vi "ReadTCPIP.vi"(3 "error in":errorcluster, 4 "TCP Timeout":i32=500, 5 "bytes to read":i32=-1, 6 "connection ID":refnum<k5>) -> (0 "errorout":errorcluster, 1 "String":string, 2 "connection ID Out":refnum<k5>)   [LabVIEW 2016]
doc: "Reads a message in from a server"
panel:
  # "-1 means read until a blank line"
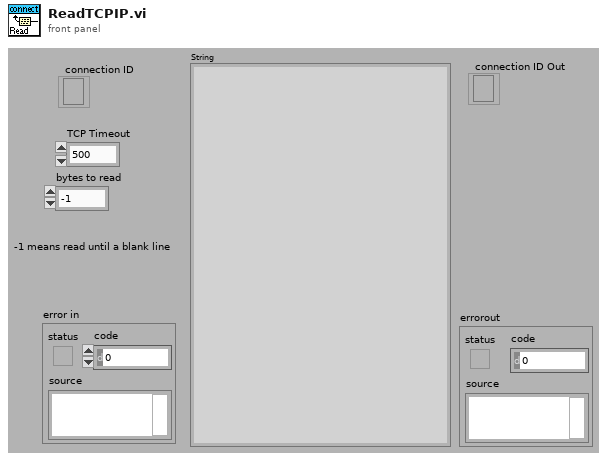
[diagram p1: front panel]
types:
  T1 = enum16{"Standard", "Buffered", "CRLF", "Immediate"}
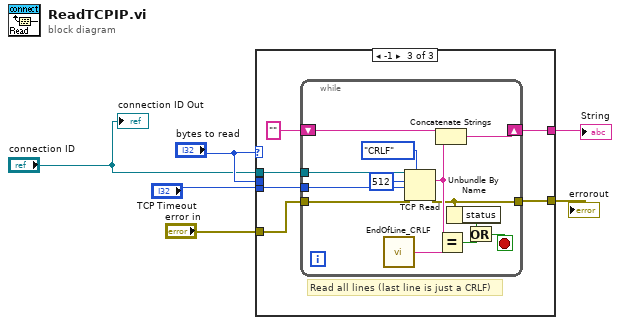
[diagram p0: block diagram]
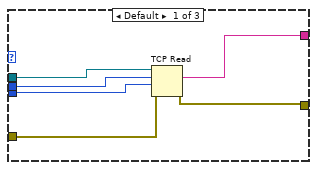
[diagram p2: hidden frame]
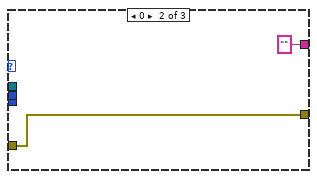
[diagram p3: hidden frame]
diagram:
  n1 = case shown="-1" "bytes to read" {
    tunnel: [w7 "" ("data out") w19] -> w6
    tunnel: [w8 w14 w18] -> w3
    tunnel: "connection ID" -> [w12 _ w17]
    tunnel: "error in" -> [w9 w14 w16]
    tunnel: "TCP Timeout" -> [w10 _ w15]
    tunnel: "bytes to read" -> [w11 _ _]
    frame Default {
      n2 = TCP Read(connection ID=w12, bytes to read=w11, error in (no error)=w9, 9:w10) -> (data out=w7:string, error out=w8:errorcluster)  [unwired: 2 out]
    }
    frame 0 {
    }
    frame -1 {
      # "Read all lines (last line is just a CRLF)"
      n3 = while {
        tunnel: w17 -> [w33]
        tunnel: w16 -> [w32]
        tunnel: [w26] -> w18
        shift-right: [w30] -> w19
        shift-left: "" -> [w31]
        tunnel: w15 -> [w22]
        stop <- w23 stop-if-true
        n4 = call "EndOfLine_CRLF.vi"() -> ("String"=w28:string)
        n5 = TCP Read(connection ID=w33, bytes to read=512, error in (no error)=w32, 7:T1."CRLF" ("mode (standard)"), 9:w22) -> (data out=w27:string, error out=w26:errorcluster)  [unwired: 1 out]
        n6 = Concatenate Strings(w31, w27) -> (w30:string)
        n7 = Equal?(x=w27, y=w28) -> (x = y?=w25:bool)
        n8 = Unbundle By Name(w26) -> ("status"=w24:bool)
        n9 = Or(x=w24, y=w25) -> (x .or. y?=w23:bool)
      }
    }
  }
  "String" <- w6
  "errorout" <- w3
  "connection ID Out" <- "connection ID"
